vi "Mono camera test.vi"() -> ()   [LabVIEW 2024]
uses:
  <vilib>/Platform/TimedLoop/XDataNode/timing_clust.ctl
  <vilib>/Platform/TimedLoop/XDataNode/nitl_modes.ctl
  <vilib>/Platform/TimedLoop/XDataNode/wakeup.ctl
  <vilib>/vision/driver/IMAQdx.llb/IMAQdx Buffer Number Mode.ctl
  <vilib>/userDefined/High Color/IMAQdx.ctl
  <vilib>/platform/TimedLoop/XDataNode/XDataNode.xnode
  <vilib>/vision/driver/NI_Vision_Acquisition_Software.lvlib
  <vilib>/Platform/TimedLoop/XDataNode/XDNodeRunTimeDep.lvlib
  <vilib>/vision/NI_Vision_Development_Module.lvlib
panel:
  out "appended array":sgl[][](array[numeric])
  in  "Pixel Y":dbl
  in  "Pixel X":dbl
  out "Image":T1(plugin-control)
  out "Pixel Value (U8)":u8
  out "Array 3":sgl[](array[numeric])
  in  "stop 2":bool
  out "Particle Measurements (Pixels) (Particle Analysis 1)":dbl[][](array[numeric]) format="%.2f"
  out "Loop iterations":i32
  out "Number of Particles (Data from objects)":i32
  out "error out":errorcluster
  out "File-name":path
  out "appended path":path
  in  "stop":bool
  out "Image Out":T1(plugin-control)
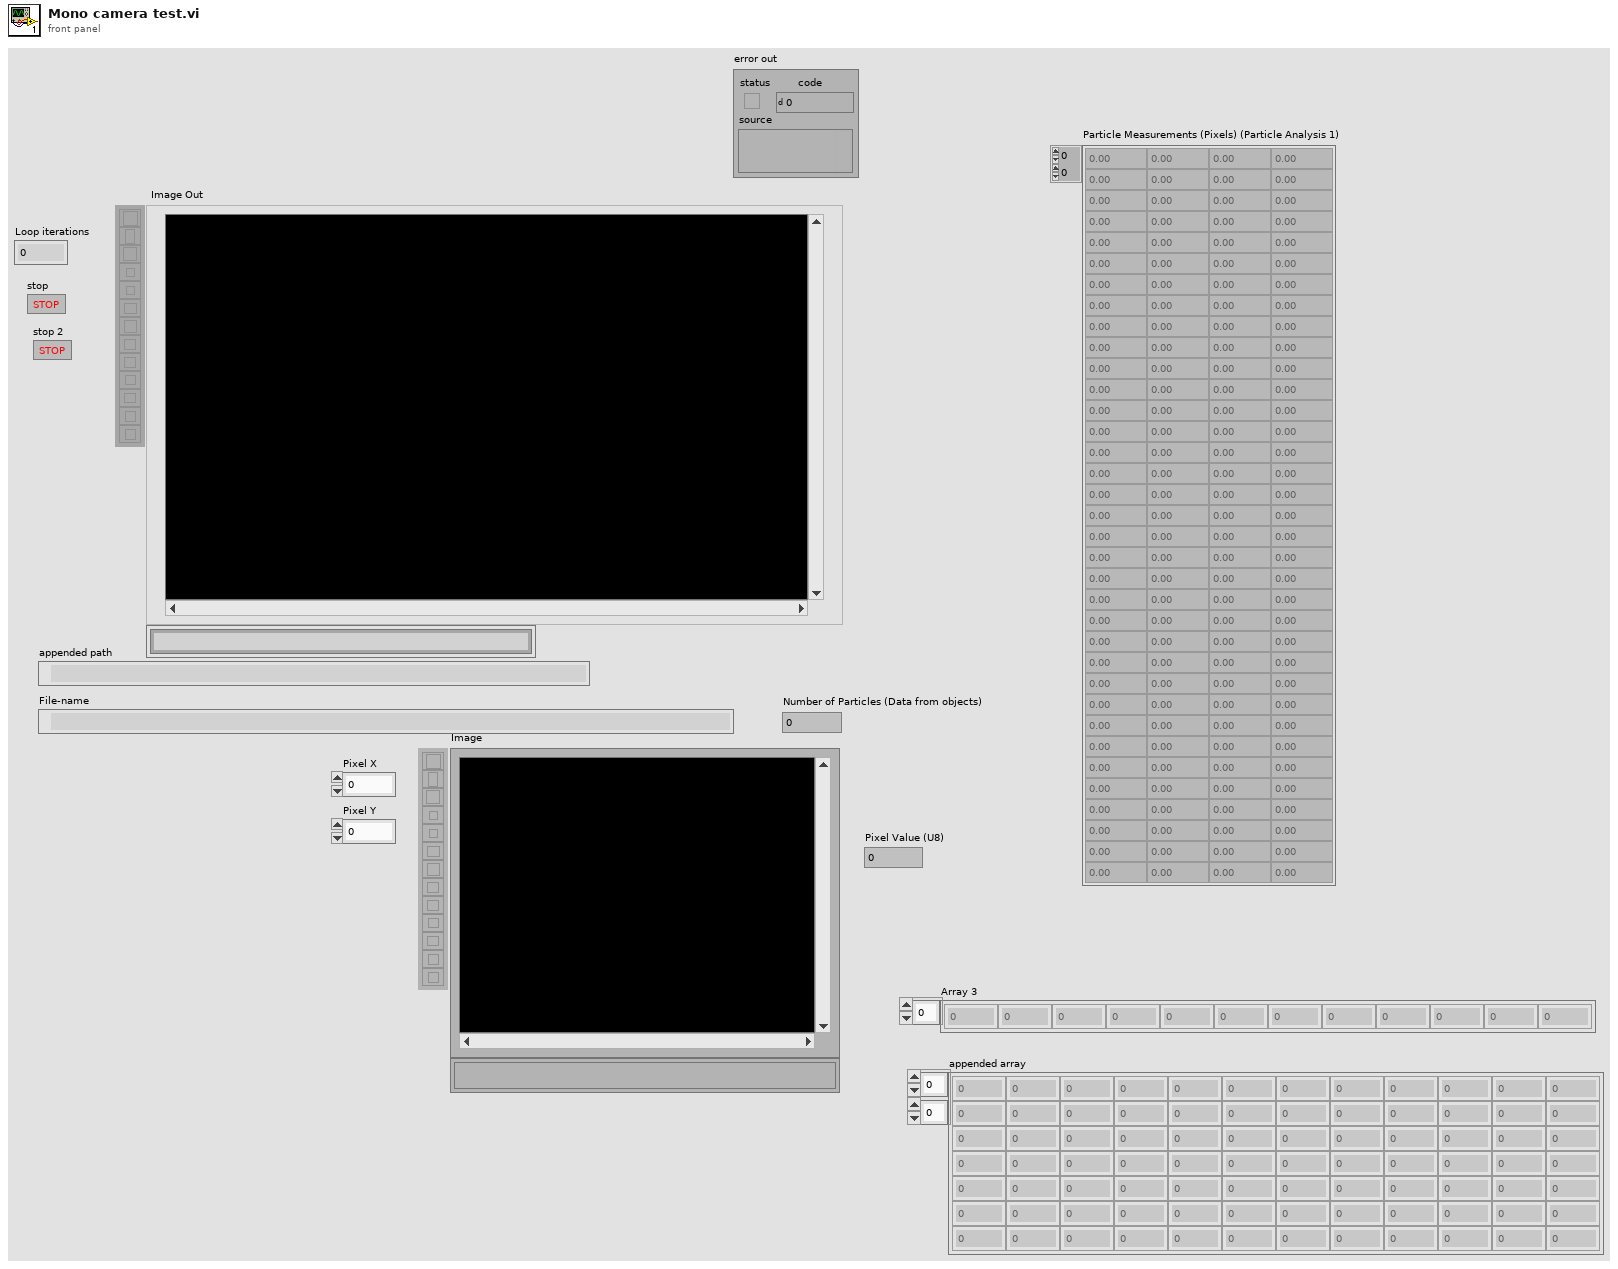
[diagram p1: front panel]
types:
  T1 = typedef "IMAQ Image.ctl" = refnum<image>
  T2 = typedef "Image Type" = u32
  T3 = typedef "IMAQdx.ctl" = refnum<k21>
  T4 = cluster{"Type":u32, "Version":u32, "Flags":u32, "SerialNumberHigh":u32, "SerialNumberLow":u32, "BusType":u32, "InterfaceName":string, "VendorName":string, "ModelName":string, "CameraFileName":string, "CameraAttributeURL":string}[]
  T5 = typedef "XDNodeRunTimeDep.lvlib/timing_clust.ctl" = cluster{"Expected End [f-1]":u64, "Actual End [f-1]":u64, "Finished Late? [f-1]":bool, "Expected End [i-1]":u64, "Actual End [i-1]":u64, "Finished Late? [i-1]":bool, "Expected Start [i]":u64, "Actual Start [i]":u64, "Expected Start [f]":u64, "Actual Start [f]":u64, "Source Name":string, "Structure Name":string, "Period":i64, "Deadline":i64, "Offset":i64, "Start":i64, "Priority":i32, "Timeout":i32, "Mode":T6, "Wakeup Reason":T7, "Error":errorcluster, "Source Type":string, "Secondary Source Type":string, "Global End Time":u64, "Global Start Time":u64, "Frame Duration":u64, "Iteration Duration":u64, "Assigned CPU":i32, "I/O Scan Engine Mode":u32}
  T6 = typedef "XDNodeRunTimeDep.lvlib/nitl_modes.ctl" = enum32{"No Change", "Process missed periods, maintain original phase", "Discard missed periods, maintain original phase", "Process missed periods, ignore original phase", "Discard missed periods, ignore original phase"}
  T7 = typedef "XDNodeRunTimeDep.lvlib/wakeup.ctl" = enum32{"Normal", "Aborted", "Asynchronous wakeup", "Timing source error", "Timed loop error", "Timeout"}
  T8 = typedef "NI_Vision_Acquisition_Software.lvlib/IMAQdx Buffer Number Mode.ctl" = enum32{"Next", "Last", "Buffer Number", "Every", "Last New"}
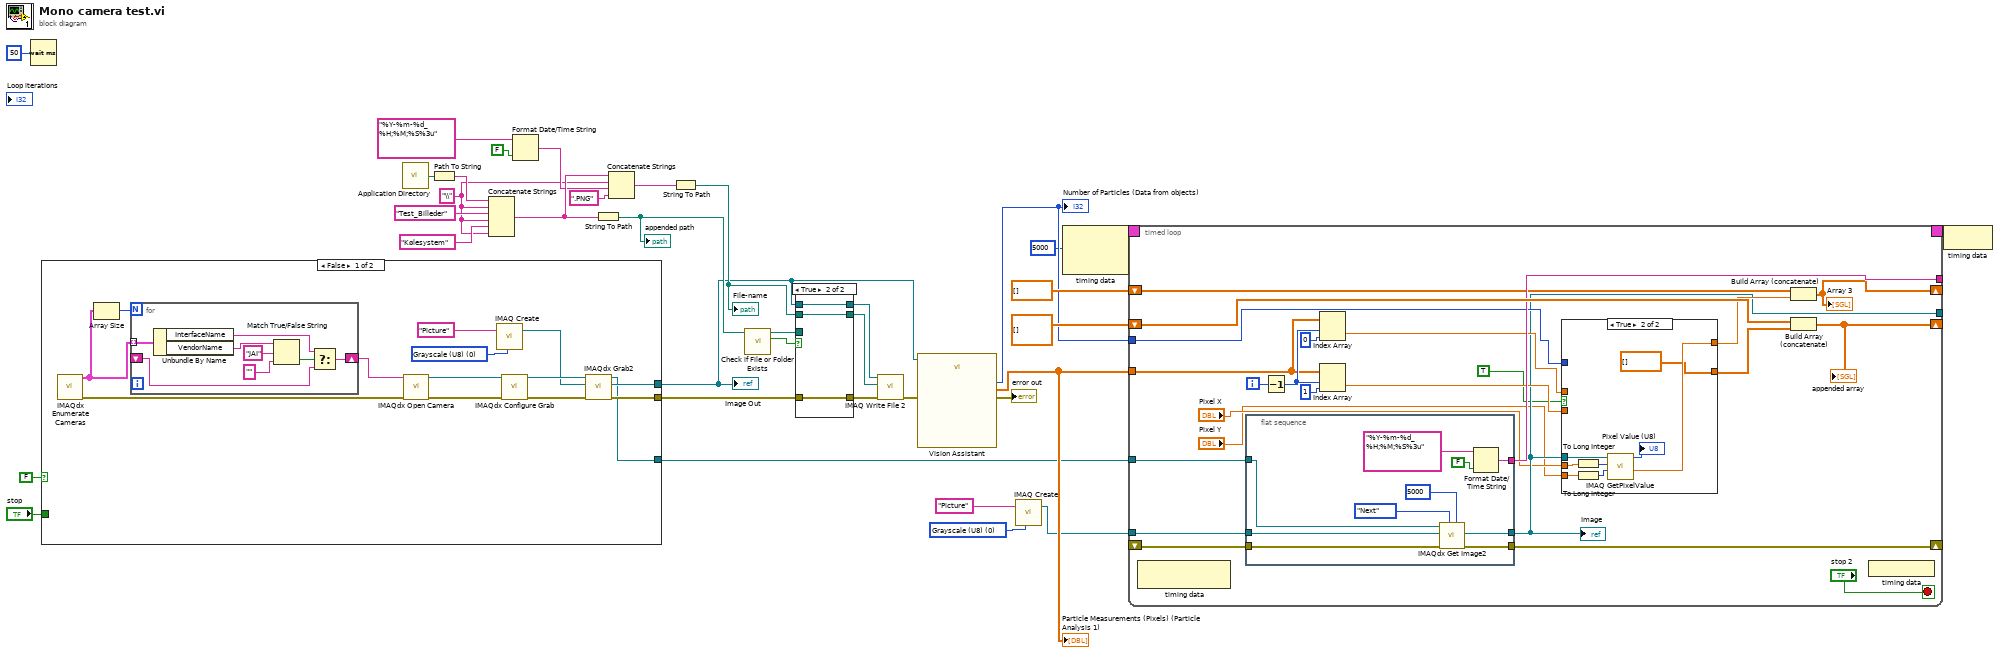
[diagram p0: block diagram]
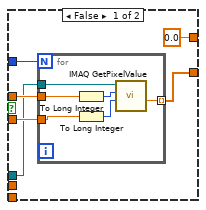
[diagram p2: hidden frame]
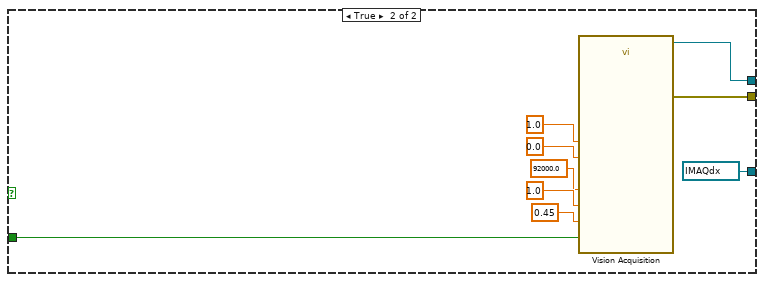
[diagram p3: hidden frame]
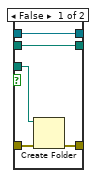
[diagram p4: hidden frame]
diagram:
  w5 = T2 0 items=["Grayscale (U8)", "Grayscale (I16)", "Grayscale (SGL)", "Complex (CSG)", "RGB (U32)", "HSL (U32)", "RGB (U64)", "Grayscale (U16)"] ("Image Type")
  w15 = "\\" ("string")
  n1 = Wait (ms)(milliseconds to wait=u32 50) -> ()  [unwired: 1 out]
  n2 = case shown="False" FALSE {
    tunnel: [w38 w66] -> w19
    tunnel: [w40 w60] -> w14
    tunnel: "stop" -> [_ w61]
    tunnel: [w37 T3 "cam5" ("Session Out")] -> w2
    frame False {
      w41 = T2 0 items=["Grayscale (U8)", "Grayscale (I16)", "Grayscale (SGL)", "Complex (CSG)", "RGB (U32)", "HSL (U32)", "RGB (U64)", "Grayscale (U16)"] ("Image Type")
      n3 = call <vilib>:"IMAQdx Enumerate Cameras.vi"() -> ("error out"=w39:errorcluster, "Camera Information Array"=w49:T4)  [unwired: 10 in]
      n4 = Array Size(array=w49) -> (size(s)=w50:i32)
      n5 = for {
        N: w50 -> [_]
        tunnel: w49 -> [w58] mode=indexing
        shift-right: [w56] -> w48
        shift-left: _ -> [w51]
        n6 = Unbundle By Name(w58) -> ("InterfaceName"=w57:string, "VendorName"=w55:string)
        n7 = Match True/False String(2:"" ("false string"), 3:"JAI" ("true string"), 4:w55) -> (0:w52:bool)  [unwired: 1 out]
        n8 = Select(t=w57, s=w52, f=w51) -> (s? t:f=w56:string)
      }
      n9 = call <vilib>:"IMAQdx Open Camera.vi"("error in"=w39, "Session In"=w48) -> ("error out"=w47:errorcluster, "Session Out"=w46:T3)  [unwired: 8 in]
      n10 = call "IMAQ Create"("Image Name"="Picture", "Image Type"=w41) -> ("New Image"=w43:T1)  [unwired: 3 in, 1 out]
      n11 = call <vilib>:"IMAQdx Configure Grab.vi"("error in"=w47, "Session In"=w46) -> ("error out"=w44:errorcluster, "Session Out"=w45:T3)  [unwired: 8 in]
      n12 = call <vilib>:"IMAQdx Grab2.vi"("error in"=w44, "Image In"=w43, "Session In"=w45) -> ("error out"=w38:errorcluster, "Image Out"=w40:T1, "Session Out"=w37:T3)  [unwired: 5 in, 1 out]
    }
    frame True {
      n13 = call "Vision Acquisition"("AcquisitionFrameRate"=1.0, "ExposureTime"=92000.0, "Gain"=1.0, "BlackLevel"=0.0, "Gamma"=0.45, "Stop (F)"=w61) -> ("Image Out"=w60:T1, "error out"=w66:errorcluster)  [unwired: 19 in, 1 out]
    }
  }
  "Image Out" <- w14
  n14 = call <vilib>:"Application Directory.vi"() -> ("Application Directory"=w33:path)
  n15 = Path To String(path=w33) -> (string=w32:string)
  n16 = Concatenate Strings(w32, w15, "Test_Billeder" ("string"), w15, "Kølesystem" ("string"), w15) -> (w27:string)
  n17 = Format Date/Time String(time format string (%c)="%Y-%m-%d_%H;%M;%S%3u", UTC format=FALSE) -> (date/time string=w24:string)  [unwired: 1 in]
  n18 = String To Path(string=w27) -> (path=w30:path)
  "appended path" <- w30
  n19 = Concatenate Strings(w27, w15, w24, ".PNG" ("string")) -> (w26:string)
  n20 = String To Path(string=w26) -> (path=w22:path)
  "File-name" <- w22
  n21 = call <vilib>:"Check if File or Folder Exists.vi"("path"=w30) -> ("file or folder exists?"=w28:bool, "dup path"=w29:path)  [unwired: 8 in, 1 out]
  n22 = case shown="True" w28 {
    tunnel: w29 -> [w72 _]
    tunnel: [w71 w75] -> w31
    tunnel: w14 -> [w71 w75]
    tunnel: w22 -> [w70 w74]
    tunnel: [w70 w74] -> w21
    tunnel: w19 -> [w69 w73]
    tunnel: [w68 w73] -> w18
    frame False {
      n23 = Create Folder(path (use dialog)=w72, error in=w69) -> (error out=w68:errorcluster)  [unwired: 1 in, 2 out]
    }
    frame True {
    }
  }
  n24 = call-poly "IMAQ Write File 2"("error in (no error)"=w18, "File Path"=w21, "Image"=w31) -> ("error out"=w17:errorcluster)  [unwired: 7 in, 1 out]
  n25 = call "Vision Assistant"("Image In"=w14, "error in"=w17) -> ("Number of Particles (Particle Analysis 1)"=w7:i32, "Particle Measurements (Pixels) (Particle Analysis 1)"=w6:dbl[][], "error out"=→"error out":errorcluster)  [unwired: 20 in, 3 out]
  "Number of Particles (Data from objects)" <- w7
  "Particle Measurements (Pixels) (Particle Analysis 1)" <- w6
  n26 = call "IMAQ Create"("Image Name"="Picture", "Image Type"=w5) -> ("New Image"=w3:T1)  [unwired: 3 in, 1 out]
  n27 = node-c288(i64 5000 ("Period")) -> (w11:T5)  [unwired: 1 in]
  n28 = timed-loop {
    shift-right: [w98] -> _
    shift-left: _ -> [w99]
    timing: w11 -> [_]
    timing-out: [_] -> w10
    shift-right: [w77] -> _
    shift-left: sgl[][] [] -> [w93]
    tunnel: [w83] -> _
    tunnel: [w92] -> _
    shift-right: [w89] -> _
    shift-left: sgl[] [] -> [w90]
    tunnel: w7 -> [w86]
    tunnel: w6 -> [w88]
    tunnel: w3 -> [w79]
    tunnel: w2 -> [w78]
    i -> [w95]
    stop <- "stop 2" stop-if-true
    n29 = node-c288() -> ()  [unwired: 1 in, 1 out]
    n30 = flat-sequence {
      tunnel: w99 -> [w127]
      tunnel: [w126] -> w98
      tunnel: [w125] -> w83
      tunnel: [w122] -> w92
      tunnel: w79 -> [w121]
      tunnel: w78 -> [w120]
      frame #0 {
        n31 = call <vilib>:"IMAQdx Get Image2.vi"("Timeout (ms)"=5000, "Buffer Number Mode (Next)"=IMAQdx_Buffer_Number_Mode."Next", "error in"=w127, "Image In"=w121, "Session In"=w120) -> ("error out"=w126:errorcluster, "Image Out"=w125:T1)  [unwired: 3 in, 2 out]
        n32 = Format Date/Time String(time format string (%c)="%Y-%m-%d_%H;%M;%S%3u", UTC format=FALSE) -> (date/time string=w122:string)  [unwired: 1 in]
      }
    }
    n33 = Decrement(x=w95) -> (x-1=w94:i32)
    n34 = Index Array(array=w88, index (row)=w94, index (col)=0 ("disabled index (col)")) -> (element=w85:dbl)
    n35 = Index Array(array=w88, index (row)=w94, index (col)=1) -> (element=w84:dbl)
    n36 = case shown="True" TRUE {
      tunnel: w83 -> [w100 w119]
      tunnel: [sgl 0.0 ("Pixel Value (Float)") w118] -> w91
      tunnel: w86 -> [w105 _]
      tunnel: w85 -> [w104 _]
      tunnel: w84 -> [w103 _]
      tunnel: [w102 sgl[] []] -> w76
      tunnel: "Pixel X" -> [_ w113]
      tunnel: "Pixel Y" -> [_ w112]
      frame False {
        n37 = for {
          N: w105 -> [_]
          tunnel: [w111] -> w102 mode=indexing
          tunnel: w104 -> [w108]
          tunnel: w103 -> [w107]
          tunnel: w100 -> [w106]
          n38 = To Long Integer(number=w108) -> (32bit integer=w110:i32)
          n39 = To Long Integer(number=w107) -> (32bit integer=w109:i32)
          n40 = call "IMAQ GetPixelValue"("Image"=w106, "X Coordinate"=w110, "Y Coordinate"=w109) -> ("Pixel Value (Float)"=w111:sgl)  [unwired: 3 in, 4 out]
        }
      }
      frame True {
        n41 = To Long Integer(number=w113) -> (32bit integer=w117:i32)
        n42 = To Long Integer(number=w112) -> (32bit integer=w116:i32)
        n43 = call "IMAQ GetPixelValue"("Image"=w119, "X Coordinate"=w117, "Y Coordinate"=w116) -> ("Pixel Value (U8)"=→"Pixel Value (U8)":u8, "Pixel Value (Float)"=w118:sgl)  [unwired: 3 in, 3 out]
      }
    }
    n44 = Build Array (concatenate)(w90, w91) -> (w89:sgl[])
    "Array 3" <- w89
    n45 = Build Array (concatenate)(w93, w76) -> (w77:sgl[][])
    "appended array" <- w77
    n46 = node-c288() -> ()  [unwired: 1 out]
    "Image" <- w83
  }
  n47 = node-c288(w10) -> ()
